vi "Align Decide.vi"(10 "Right Ping":dbl, 11 "Left Ping":dbl) -> (3 "Next Step":T1)   [LabVIEW 2014]
uses:
  Common Code/Inner Roller States.ctl
  Robot Global Data.vi
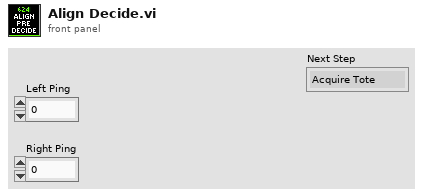
[diagram p1: front panel]
types:
  T1 = typedef "Inner Roller States.ctl" = enum16{"Acquire Tote", "Absorb Tote", "Turn Tote Right", "Turn Tote Left"}
  T2 = typedef "Dashboard Control Data.ctl" = cluster{"Cam Exposure":dbl, "Go to angle":dbl, "Steer PID Gains":cluster{"proportional gain (Kc)":dbl, "integral time (Ti, min)":dbl, "derivative time (Td, min)":dbl}, "Steer PID output Range":cluster{"output high":dbl, "output low":dbl}, "Pressure m \nValue":dbl, "Pressure b \nValue":dbl, "Strafe Timer\nWait":dbl, "Roller Command Cluster ":T3, "Elevator":T4, "Strafe Correct min X":dbl, "IMU Enable":bool, "Encoder Control":T6}
  T3 = typedef "Roller Control.ctl" = cluster{"Intake Speed":dbl, "Turn In Speed":dbl, "Unload Speed":dbl, "Turn Out Speed":dbl, "Ping Align Tolerance":dbl, "Tote Range Threshold":dbl, "Right Pot 0":dbl, "Pot Threshold":dbl, "Left Pot 0":dbl, "Manual 0s?":bool, "Right Pot Scale":dbl, "Left Pot Scale":dbl, "0 wait time":i32, "Zero Pots":bool}
  T4 = typedef "Elevator DB Control.ctl" = cluster{"PID Output Range":cluster{"output high":dbl, "output low":dbl}, "PID gains":cluster{"proportional gain (Kc)":dbl, "integral time (Ti, min)":dbl, "derivative time (Td, min)":dbl}, "Height Tolerance":dbl, " Encoder Constant":dbl, "Safe Mode Max Speed":dbl, "Eject Time":dbl, "Encoder Filter?":bool, "Zeroing Speed":dbl, "Presets":T5}
  T5 = typedef "Elevator Presets.ctl" = cluster{"Hold Tote":dbl, "Hold Trashcan":dbl, "Pickup 2 w/ Tote":dbl, "Pickup 2 w/ Trashcan":dbl, "Pickup 3 w/ Tote":dbl, "Pickup 3 w/ Trashcan":dbl, "Bottom":dbl, "Pickup 1 w/ Tote":dbl, "Pickup Trashcan":dbl, "Pickup 1 w/ Trashcan":dbl, "Eject":dbl}
  T6 = typedef "Encoder Control.ctl" = cluster{"Left Tick Constant":dbl, "Right Tick Constant":dbl, "Center Tick Constant":dbl, "Reset?":bool}
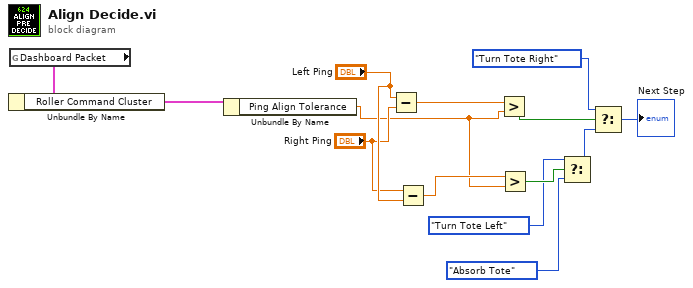
[diagram p0: block diagram]
diagram:
  n1 = global read "Robot Global Data.vi" "Dashboard Packet"() -> (w5:T2)
  n2 = Unbundle By Name(w5) -> ("Roller Command Cluster"=w4:T3)
  n3 = Unbundle By Name(w4) -> ("Ping Align Tolerance"=w1:dbl)
  n4 = Subtract(x="Left Ping", y="Right Ping") -> (x-y=w14:dbl)
  n5 = Subtract(x="Right Ping", y="Left Ping") -> (x-y=w13:dbl)
  n6 = Greater?(x=w14, y=w1) -> (0:w11:bool)
  n7 = Greater?(x=w13, y=w1) -> (0:w10:bool)
  n8 = Select(t=Inner_Roller_States."Turn Tote Left", s=w10, f=Inner_Roller_States."Absorb Tote") -> (s? t:f=w12:T1)
  n9 = Select(t=Inner_Roller_States."Turn Tote Right", s=w11, f=w12) -> (s? t:f=→"Next Step":T1)
